vi "Do.vi"(8 "error in":errorcluster, 10 "Actor in":refnum<class "Actor.lvclass">, 11 "Change Meerstetter Power":refnum<class "Change Meerstetter Power.lvclass">) -> (0 "error out":errorcluster, 2 "Actor out":refnum<class "Actor.lvclass">)   [LabVIEW 2014, in "Meerstetter Lib.lvlib" / "Change Meerstetter Power.lvclass"]
doc: "(<B>Filename</B>: Actor Framework.lvlib:Message.lvclass:Do.vi)\n\nDefines what a message does when it is received by an actor. Generally, a message instructs an actor to invoke one of its methods. By default, this method does nothing. A child class must override it to define behavior. Create a child class by using the Actor Framework Message Maker dialog box."
uses:
  Change Meerstetter Power.lvclass
  <vilib>/ActorFramework/Actor/Actor.lvclass
  reusable/DAQ Device/Device/Device.lvclass
  Meerstetter TEC.lvclass
  reusable/DAQ Device/Device/Device.lvclass/Device.ctl
  SuperActor/SuperActor.lvclass/SuperActor.ctl
  Change Meerstetter Power.lvclass/Change Meerstetter Power.ctl
  reusable/DAQ Device/Device/Read Configurable Device.vi
  SuperActor/Read CVT Session.vi
  SuperActor/Read ID.vi
  Configurable Device/Configurable Device.lvclass
  <userlib>/_Session Fwk/Session - Root.lvclass
  reusable/Session APIs/CVT/CVT.lvclass
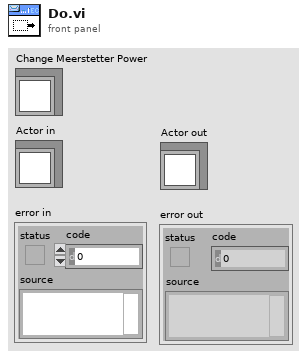
[diagram p1: front panel]
types:
  T1 = typedef "Session - Root.lvclass/Session Handle.ctl" = refnum<data-value>
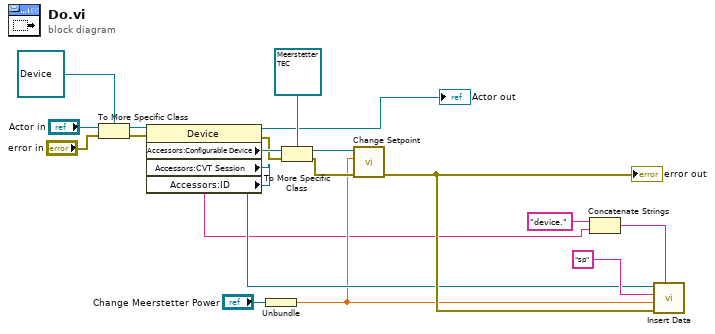
[diagram p0: block diagram]
diagram:
  n1 = To More Specific Class(target class=refnum<class "Device.lvclass"> refnum ("DAQ Device.lvlib:Device"), reference="Actor in", error in="error in") -> (specific class reference=w15:refnum<class "Device.lvclass">, error out=w16:errorcluster)
  n2 = property class="Device"(reference=w15, error in=w16) -> (reference out=→"Actor out":refnum<class "Device.lvclass">, error out=w13:errorcluster, "Accessors:Configurable Device"=w14:refnum<class "Configurable Device.lvclass">, "Accessors:CVT Session"=w3:T1, "Accessors:ID"=w1:string)
  n3 = Unbundle("Change Meerstetter Power") -> (w2:sgl)
  n4 = To More Specific Class(target class=refnum<class "Meerstetter TEC.lvclass"> refnum ("Meerstetter Lib.lvlib:TEC 1090"), reference=w14, error in=w13) -> (specific class reference=w11:refnum<class "Meerstetter TEC.lvclass">, error out=w9:errorcluster)
  n5 = call-dynamic "Change Setpoint.vi"("error in"=w9, "Setpoint"=w2, "Meerstetter TEC in"=w11) -> ("error out"=w4:errorcluster)  [unwired: 7 in, 1 out]
  "error out" <- w4
  n6 = Concatenate Strings("device." ("string"), w1) -> (w6:string)
  n7 = call "Insert Data.vi"("Group"=w6, "error in"=w4, "Data"=w2, "tag"="sp", "CVT Session In"=w3) -> ()  [unwired: 5 in, 2 out]
